vi "Select Symbol.vi"(11 "Hierarchy":string[](array[string])) -> (3 "Symbol ID":string)   [LabVIEW 2020, in "Project Tree.lvlib" / "Project Tree Map.lvclass"]
uses:
  Project Tree Map.lvclass
  Project Tree Map.lvclass/Project Tree Map.ctl
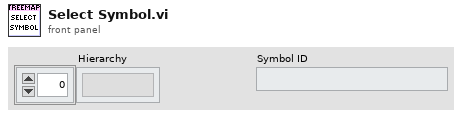
[diagram p1: front panel]
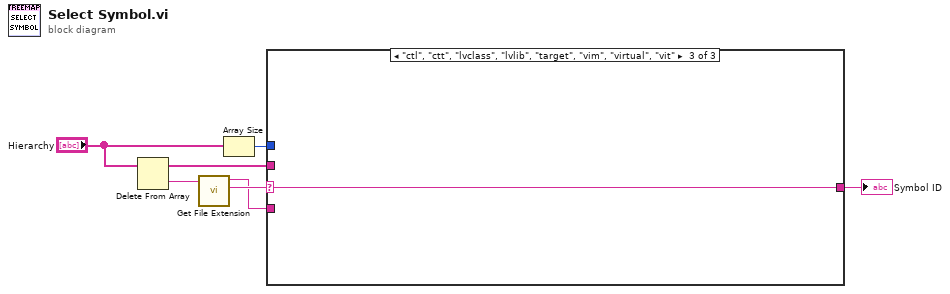
[diagram p0: block diagram]
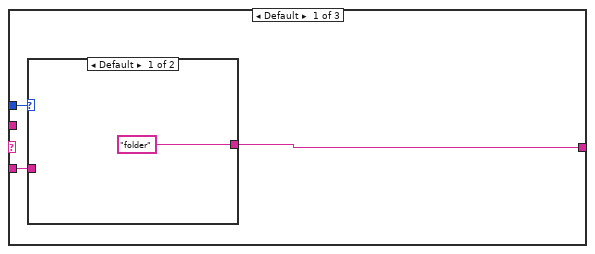
[diagram p2: hidden frame]
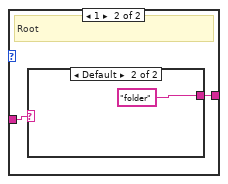
[diagram p3: hidden frame]
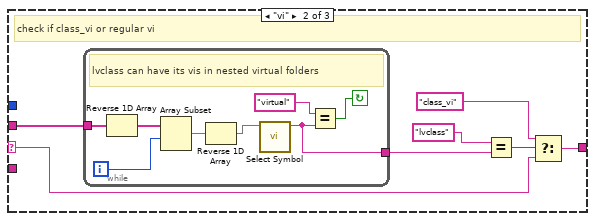
[diagram p5: hidden frame]
diagram:
  n1 = Delete From Array(array="Hierarchy") -> (deleted portion=w4:string, array with subset deleted=w1:string[])  [unwired: 2 in]
  n2 = call "Get File Extension.vi"("Filename"=w4) -> ("Lowercase Extension"=w3:string, "Filename without Extension"=w2:string)  [unwired: 9 in]
  n3 = Array Size(array="Hierarchy") -> (size(s)=w6:i32)
  n4 = case shown="\"ctl\", \"ctt\", \"lvclass\", \"lvlib\", \"target\", \"vim\", \"virtual\", \"vit\"" w3 {
    selector: w3 -> [_ w18 w31]
    tunnel: [w10 w17 w31] -> w7
    tunnel: w2 -> [w9 _ _]
    tunnel: w6 -> [w8 _ _]
    tunnel: w1 -> [_ w22 _]
    frame Default {
      n5 = case shown="Default" w8 {
        tunnel: ["folder" w13] -> w10
        tunnel: w9 -> [_ w12]
        frame Default {
        }
        frame 1 {
          # "Root"
          n6 = case shown="Default" w12 {
            selector: w12 -> [w14 _]
            tunnel: [w14 "folder"] -> w13
            frame "My Computer" {
            }
            frame Default {
            }
          }
        }
      }
    }
    frame "vi" {
      # "check if class_vi or regular vi"
      n7 = while {
        tunnel: w22 -> [w27]
        tunnel: [w29] -> w21
        i -> [w25]
        stop <- w28 continue-if-true
        # "lvclass can have its vis in nested virtual folders"
        n8 = Reverse 1D Array(array=w27) -> (reversed array=w24:string[])
        n9 = Array Subset(array=w24, index=w25) -> (w26:string[])  [unwired: 1 in]
        n10 = Reverse 1D Array(array=w26) -> (reversed array=w23:string[])
        n11 = call "Select Symbol.vi"("Hierarchy"=w23) -> ("Symbol ID"=w29:string)  [unwired: 10 in]
        n12 = Equal?(x="virtual", y=w29) -> (x = y?=w28:bool)
      }
      n13 = Equal?(x="lvclass", y=w21) -> (x = y?=w20:bool)
      n14 = Select(t="class_vi", s=w20, f=w18) -> (s? t:f=w17:string)
    }
    frame "ctl", "ctt", "lvclass", "lvlib", "target", "vim", "virtual", "vit" {
    }
  }
  "Symbol ID" <- w7
